vi "Run.vi"(7 "Team Index":i32, 8 "Column":i32, 9 "Row":i32, 10 "View":i32[](array[numeric]) caption="View (Team Index, -1: empty)", 11 "MRM Clones In":refnum<class "MRM Clones.lvclass">) -> (0 "Replicated":refnum<class "Square.lvclass">, 1 "Direction":T1, 2 "Action":T2, 3 "Square Out":refnum<class "Square.lvclass">)   [LabVIEW 2020, in "MRM Clones.lvclass"]
uses:
  MRM Clones.lvclass
  C:/dev/IlluminatedG/sol-squarebattle/Square/Square.lvclass
  Square/Square.lvclass
  Type Defs/Action Enum.ctl
  Type Defs/Direction Enum.ctl
  MRM Clones.lvclass/MRM Clones.ctl
  SubVIs/Read-Only Globals.vi
  SubVIs/Globals (private).vi
  Common/Common.lvlib
  Type Defs/SB Type Defs.lvlib
panel:
  # "NW\nN\nNE\nE\nSE\nS\nSW\nW"
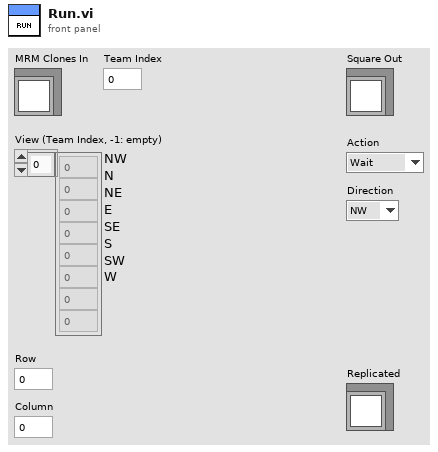
[diagram p1: front panel]
types:
  T1 = typedef "SB Type Defs.lvlib/Direction Enum.ctl" = enum16{"NW", "N", "NE", "E", "SE", "S", "SW", "W"}
  T2 = typedef "SB Type Defs.lvlib/Action Enum.ctl" = enum16{"Wait", "Move", "Attack", "Replicate"}
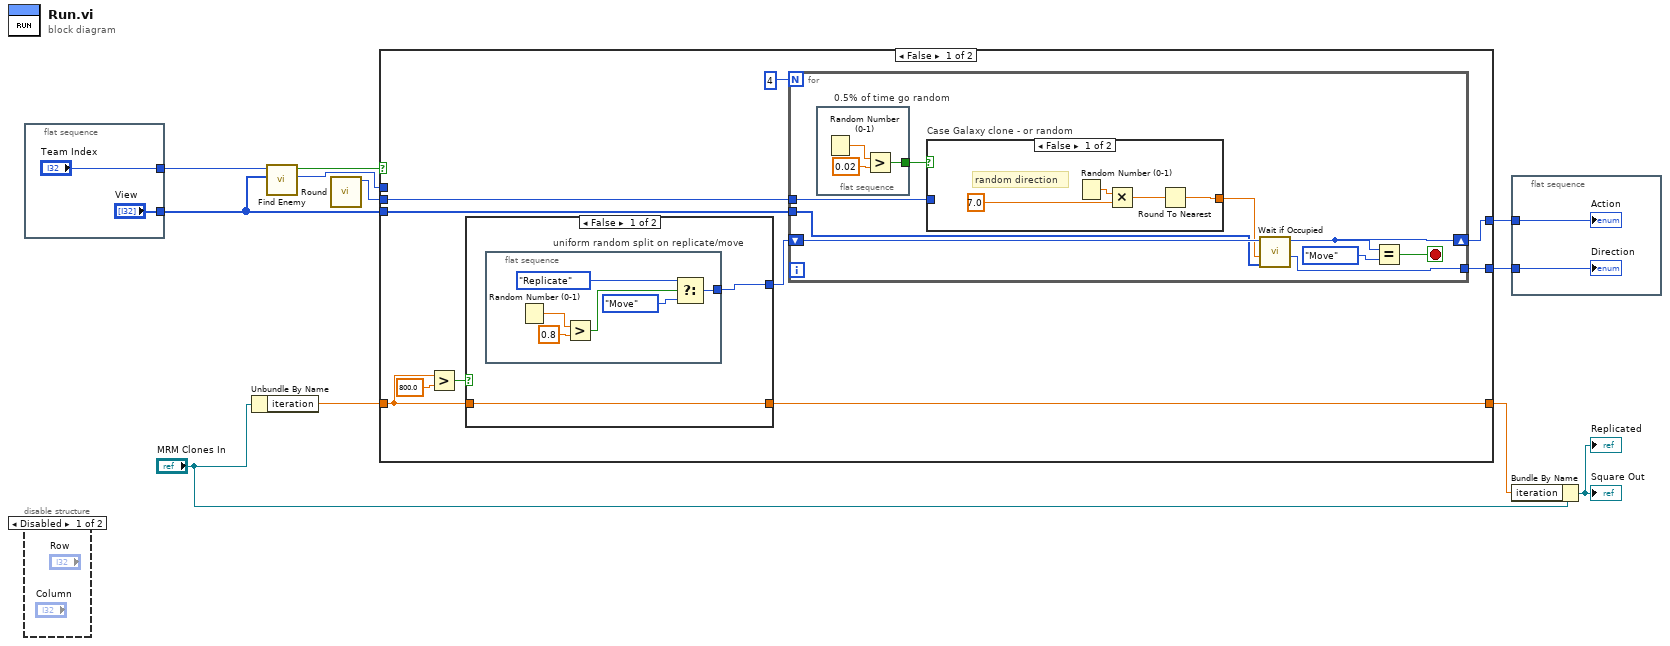
[diagram p0: block diagram]
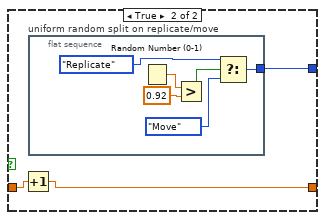
[diagram p3: hidden frame]
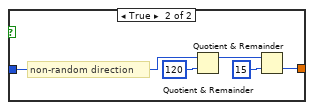
[diagram p4: hidden frame]
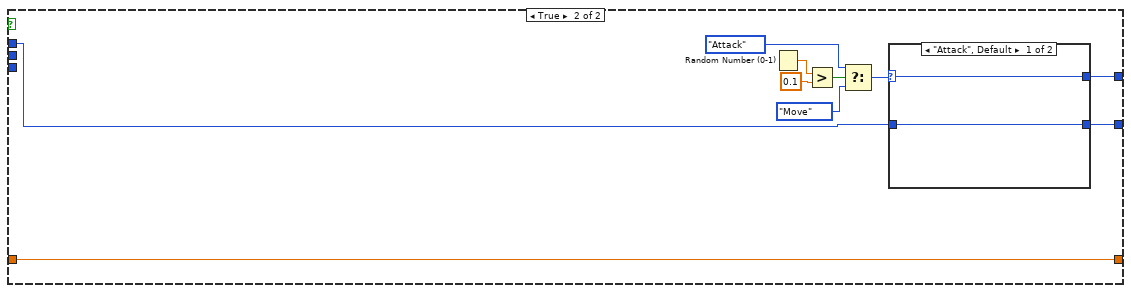
[diagram p5: hidden frame]
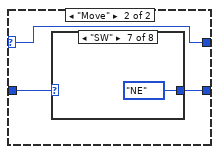
[diagram p6: hidden frame]
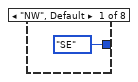
[diagram p7: hidden frame]
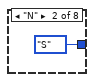
[diagram p8: hidden frame]
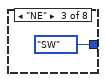
[diagram p9: hidden frame]
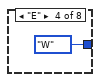
[diagram p10: hidden frame]
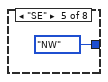
[diagram p11: hidden frame]
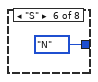
[diagram p12: hidden frame]
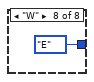
[diagram p13: hidden frame]
diagram:
  n1 = flat-sequence {
    tunnel: ["View"] -> w8
    tunnel: ["Team Index"] -> w7
    frame #0 {
    }
  }
  n2 = disable-structure shown="Disabled" {
    frame Disabled {
    }
    frame Enabled {
    }
  }
  n3 = Unbundle By Name("MRM Clones In") -> ("iteration"=w4:dbl)
  n4 = call "Find Enemy.vi"("View"=w8, "Team Index"=w7) -> ("Direction"=w10:T1, "Found Enemy?"=w11:bool)  [unwired: 7 in, 1 out]
  n5 = call "Round.vi"() -> ("Round"=w9:i32)  [unwired: 11 in]
  n6 = case shown="False" w11 {
    tunnel: [w20 w62] -> w6
    tunnel: w10 -> [_ w64]
    tunnel: [w22 w63] -> w5
    tunnel: w9 -> [w23 _]
    tunnel: w8 -> [w21 _]
    tunnel: w4 -> [w16 w71]
    tunnel: [w14 w71] -> w3
    frame False {
      n7 = Greater?(x=w16, y=800.0) -> (0:w17:bool)
      n8 = case shown="False" w17 {
        tunnel: w16 -> [w24 w33]
        tunnel: [w25 w34] -> w15
        tunnel: [w24 w32] -> w14
        frame False {
          n9 = flat-sequence "uniform random split on replicate/move" {
            tunnel: [w26] -> w25
            frame #0 {
              n10 = Random Number (0-1)() -> (number: 0 to 1=w31:dbl)
              n11 = Greater?(x=w31, y=0.8) -> (0:w29:bool)
              n12 = Select(t=Action_Enum."Replicate" ("Action"), s=w29, f=Action_Enum."Move" ("Action")) -> (s? t:f=w26:T2)
            }
          }
        }
        frame True {
          n13 = Increment(x=w33) -> (x+1=w32:dbl)
          n14 = flat-sequence "uniform random split on replicate/move" {
            tunnel: [w35] -> w34
            frame #0 {
              n15 = Random Number (0-1)() -> (number: 0 to 1=w40:dbl)
              n16 = Greater?(x=w40, y=0.92) -> (0:w38:bool)
              n17 = Select(t=Action_Enum."Replicate" ("Action"), s=w38, f=Action_Enum."Move" ("Action")) -> (s? t:f=w35:T2)
            }
          }
        }
      }
      n18 = for {
        N: 4 -> [_]
        tunnel: w23 -> [w49]
        tunnel: [w47] -> w22
        tunnel: w21 -> [w46]
        shift-right: [w43] -> w20
        shift-left: w15 -> [w48]
        stop <- w41 stop-if-true
        n19 = flat-sequence "0.5% of time go random" {
          tunnel: [w50] -> w44
          frame #0 {
            n20 = Random Number (0-1)() -> (number: 0 to 1=w52:dbl)
            n21 = Greater?(x=w52, y=0.02) -> (0:w50:bool)
          }
        }
        n22 = case "Case Galaxy clone - or random" shown="False" w44 {
          tunnel: w49 -> [_ w61]
          tunnel: [w53 w60] -> w45
          frame False {
            # "random direction"
            n23 = Random Number (0-1)() -> (number: 0 to 1=w56:dbl)
            n24 = Multiply(x=w56, y=7.0) -> (x*y=w54:dbl)
            n25 = Round To Nearest(number=w54) -> (nearest integer value=w53:dbl)
          }
          frame True {
            # "non-random direction"
            n26 = Quotient & Remainder(x=w61, y=120) -> (x-y*floor(x/y)=w57:i32)  [unwired: 1 out]
            n27 = Quotient & Remainder(x=w57, y=15) -> (floor(x/y)=w60:i32)  [unwired: 1 out]
          }
        }
        n28 = call "Wait if Occupied.vi"("View"=w46, "Direction In"=w45, "Action In"=w48) -> ("Direction Out"=w47:T1, "Action Out"=w43:T2)  [unwired: 7 in]
        n29 = Equal?(x=w43, y=Action_Enum."Move") -> (x = y?=w41:bool)
      }
    }
    frame True {
      n30 = Random Number (0-1)() -> (number: 0 to 1=w70:dbl)
      n31 = Greater?(x=w70, y=0.1) -> (0:w68:bool)
      n32 = Select(t=Action_Enum."Attack" ("Action"), s=w68, f=Action_Enum."Move" ("Action")) -> (s? t:f=w65:T2)
      n33 = case shown="\"Attack\", Default" w65 {
        selector: w65 -> [w72 w74]
        tunnel: w64 -> [w73 w76]
        tunnel: [w73 w75] -> w63
        tunnel: [w72 w74] -> w62
        frame "Attack", Default {
        }
        frame "Move" {
          n34 = case shown="\"SW\"" w76 {
            tunnel: [Direction_Enum."SE" ("Direction 2") Direction_Enum."S" ("Direction 2") Direction_Enum."SW" ("Direction 2") Direction_Enum."W" ("Direction 2") Direction_Enum."NW" ("Direction 2") Direction_Enum."N" ("Direction 2") Direction_Enum."NE" ("Direction 2") Direction_Enum."E" ("Direction 2")] -> w75
            frame "NW", Default {
            }
            frame "N" {
            }
            frame "NE" {
            }
            frame "E" {
            }
            frame "SE" {
            }
            frame "S" {
            }
            frame "SW" {
            }
            frame "W" {
            }
          }
        }
      }
    }
  }
  n35 = flat-sequence {
    tunnel: w6 -> [w86]
    tunnel: w5 -> [w85]
    frame #0 {
      "Action" <- w86
      "Direction" <- w85
    }
  }
  n36 = Bundle By Name(cluster="MRM Clones In", "iteration"=w3) -> (→"Square Out" →"Replicated":refnum<class "MRM Clones.lvclass">)
